vi "String to Magnet device cluster.vi"(11 "Magnet Device Details":string="VTRT:0:STAT:0:NICK:GRPN:BIPL:ON:MAN:HVER::FVER::SERL::ATOB:1.0:SWPR:None:SHTC:100.0:VLIM:10.00:IND:1:CLIM:10.0:ACTN:CLMP:SIG:CURR:0.0000A:PCUR:0.0000A:VOLT:0.0000V:RCST:0.0000A/m:RFST:0.0000T/m:SWHN:OFF:FSET:0.0000T:FLD:0.0000T:RFLD:1200.0000T/min:CSET:0.0000A:RCUR:1200.0000A/min:PFLD:0.0000T:SWHT:OFF:OCNF:PARA") -> (3 "Magnet PSU":T1={"Manufacturing"={"Hardware Version"="", "Firmware Version"="", "Serial Number"=""}, "Nickname"="", "Bipolar Output"="", "String"="SERS", "Current Limit"=0.0, "AtoB"=0.0, "Inductance"=0.0, "Switch Present"="", "Swh Htr Current"=0.0, "SW VLIM"=0.0, "V Trans Time"=0.0, "Magnet PSU Signals"={"Voltage"=0.0, "Current"=0.0, "Current Rate"=0.0, "Field"=0.0, "Field Rate"=0.0, "Persistant Current"=0.0, "Persistant Field"=0.0, "Target Current"=0.0, "Target Field"=0.0, "Target Current Rate"=0.0, "Target Field Rate"=0.0, "Switch Heater Status (SWHT)"="", "Switch Heater Status (SWHN)"=""}, "PSU Action"="SERS", "Status"="", "Level Limit"=0.0, "Temperature Limit"=0.0} {"Temperature Limit" format="%#.1f"; "Level Limit" format="%#.1f"; "V Trans Time" format="%#.1f"; "SW VLIM" format="%#.1f"; "Swh Htr Current" format="%#.1f"; "Inductance" format="%#.1f"; "AtoB" format="%#.1f"; "Current Limit" format="%#.1f"})   [LabVIEW 2018, in "Mercury iXX.lvlib" / "Magnet.lvlib"]
uses:
  Magnet.lvlib
  Device (Read).ctl
  Manufacturing Data.ctl
  Signals (Read).ctl
  Mercury iXX.lvlib
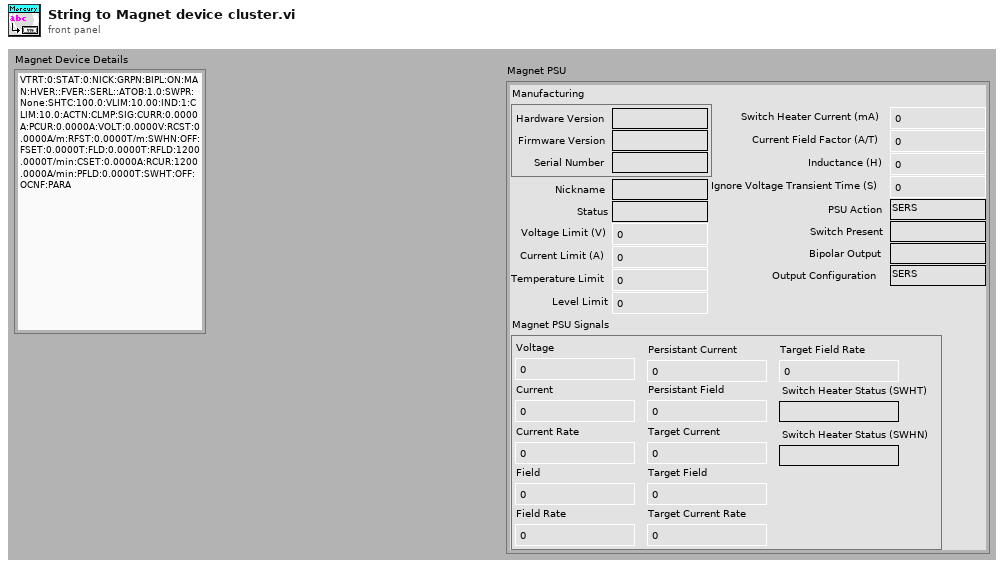
[diagram p1: front panel]
types:
  T1 = typedef "Mercury iXX.lvlib/Magnet.lvlib/Device (Read).ctl" = cluster{"Manufacturing":T2, "Nickname":string, "Bipolar Output":string, "String":string, "Current Limit":dbl, "AtoB":dbl, "Inductance":dbl, "Switch Present":string, "Swh Htr Current":dbl, "SW VLIM":dbl, "V Trans Time":dbl, "Magnet PSU Signals":T3, "PSU Action":string, "Status":string, "Level Limit":dbl, "Temperature Limit":dbl}
  T2 = typedef "Mercury iXX.lvlib/Manufacturing Data.ctl" = cluster{"Hardware Version":string, "Firmware Version":string, "Serial Number":string}
  T3 = typedef "Mercury iXX.lvlib/Magnet.lvlib/Signals (Read).ctl" = cluster{"Voltage":dbl, "Current":dbl, "Current Rate":dbl, "Field":dbl, "Field Rate":dbl, "Persistant Current":dbl, "Persistant Field":dbl, "Target Current":dbl, "Target Field":dbl, "Target Current Rate":dbl, "Target Field Rate":dbl, "Switch Heater Status (SWHT)":string, "Switch Heater Status (SWHN)":string}
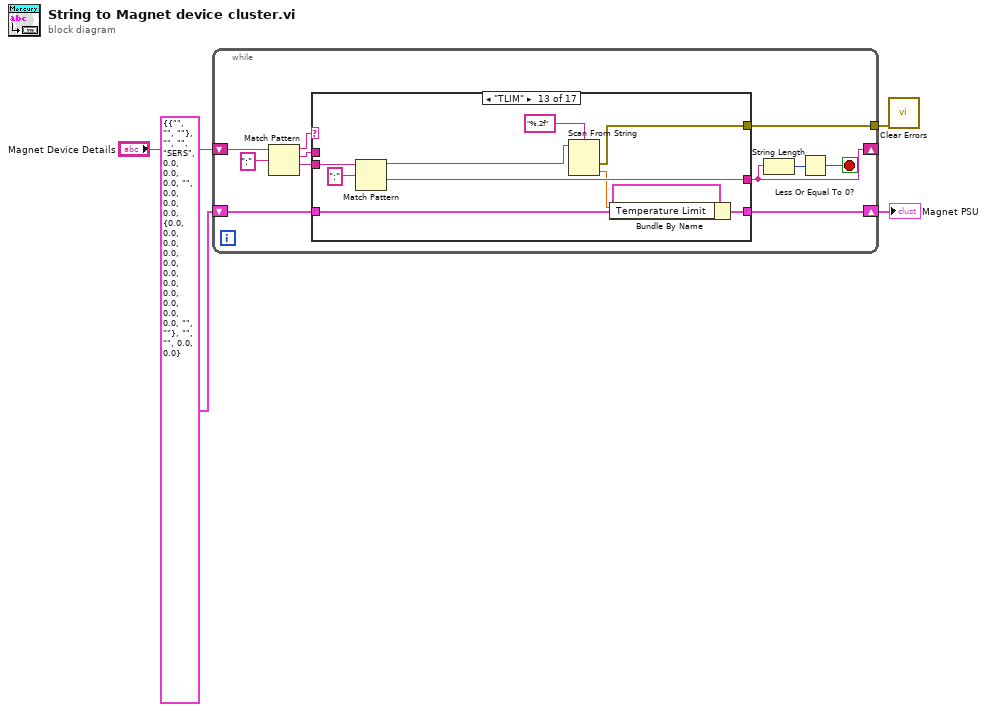
[diagram p0: block diagram]
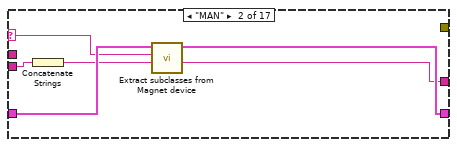
[diagram p3: hidden frame]
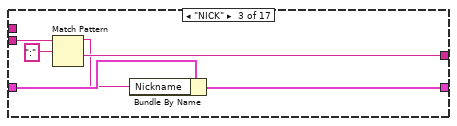
[diagram p4: hidden frame]
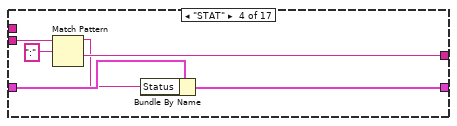
[diagram p5: hidden frame]
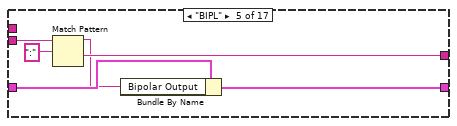
[diagram p6: hidden frame]
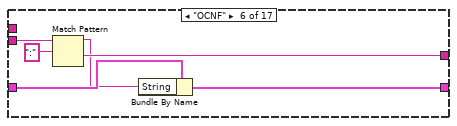
[diagram p7: hidden frame]
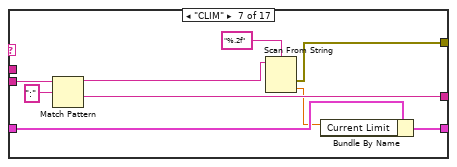
[diagram p8: hidden frame]
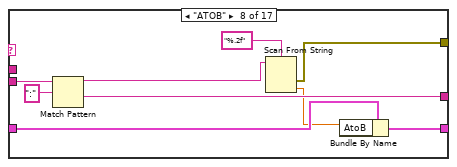
[diagram p9: hidden frame]
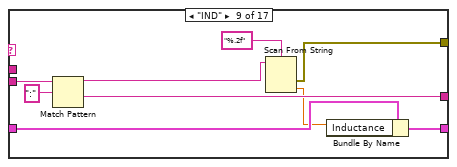
[diagram p10: hidden frame]
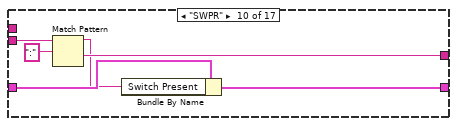
[diagram p11: hidden frame]
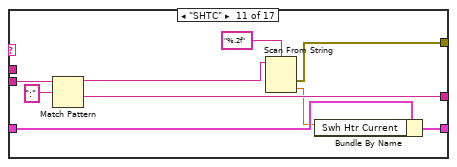
[diagram p12: hidden frame]
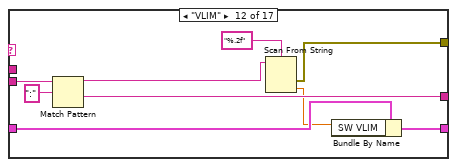
[diagram p13: hidden frame]
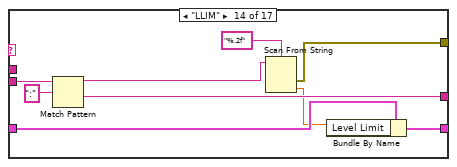
[diagram p14: hidden frame]
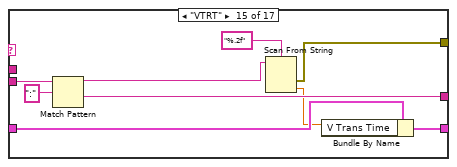
[diagram p15: hidden frame]
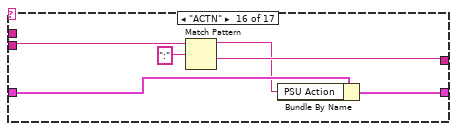
[diagram p16: hidden frame]
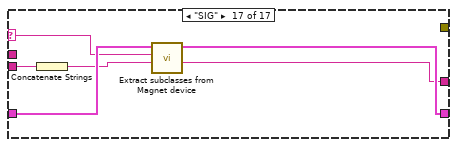
[diagram p17: hidden frame]
diagram:
  n1 = while {
    shift-right: [w11] -> w3
    shift-left: T1 {"Manufacturing"={"Hardware Version"="", "Firmware Version"="", "Serial Number"=""}, "Nickname"="", "Bipolar Output"="", "String"="SERS", "Current Limit"=0.0, "AtoB"=0.0, "Inductance"=0.0, "Switch Present"="", "Swh Htr Current"=0.0, "SW VLIM"=0.0, "V Trans Time"=0.0, "Magnet PSU Signals"={"Voltage"=0.0, "Current"=0.0, "Current Rate"=0.0, "Field"=0.0, "Field Rate"=0.0, "Persistant Current"=0.0, "Persistant Field"=0.0, "Target Current"=0.0, "Target Field"=0.0, "Target Current Rate"=0.0, "Target Field Rate"=0.0, "Switch Heater Status (SWHT)"="", "Switch Heater Status (SWHN)"=""}, "PSU Action"="", "Status"="", "Level Limit"=0.0, "Temperature Limit"=0.0} ("Magnet PSU") -> [w12]
    shift-right: [w7] -> _
    shift-left: "Magnet Device Details" -> [w14]
    tunnel: [w5] -> w1
    stop <- w6 stop-if-true
    n2 = Match Pattern(string=w14, regular expression=":") -> (before substring=w13:string, match substring=w10:string, after substring=w9:string)  [unwired: 2 out]
    n3 = case shown="\"TLIM\"" w13 {
      selector: w13 -> [_ w22 _ _ _ _ _ _ _ _ _ _ _ _ _ _ w135]
      tunnel: w10 -> [_ _ _ _ _ _ _ _ _ _ _ _ _ _ _ _ _]
      tunnel: w12 -> [w17 w23 w27 w33 w39 w45 w54 w63 w72 w78 w87 w96 w105 w114 w123 w128 w136]
      tunnel: [w17 w21 w26 w32 w38 w44 w53 w62 w71 w77 w86 w95 w104 w113 w122 w127 w133] -> w11
      tunnel: [w16 w20 w25 w31 w37 w43 w51 w60 w69 w76 w84 w93 w102 w111 w120 w129 w132] -> w7
      tunnel: w9 -> [w16 w19 w28 w34 w40 w46 w55 w64 w73 w79 w88 w97 w106 w115 w124 w130 w137]
      tunnel: [_ _ _ _ _ _ w48 w57 w66 _ w81 w90 w99 w108 w117 _ _] -> w5
      frame "", Default {
      }
      frame "MAN" {
        n4 = Concatenate Strings(w19) -> (w18:string)
        n5 = call "Extract subclasses from Magnet device.vi"("Data In"=w18, "Class"=w22, "Aux Device Settings in"=w23) -> ("Data out"=w20:string, "Aux Device Settings out"=w21:T1)  [unwired: 7 out]
      }
      frame "NICK" {
        n6 = Match Pattern(string=w28, regular expression=":") -> (before substring=w24:string, after substring=w25:string)  [unwired: 3 out]
        n7 = Bundle By Name(cluster=w27, "Nickname"=w24) -> (w26:T1)
      }
      frame "STAT" {
        n8 = Match Pattern(string=w34, regular expression=":") -> (before substring=w30:string, after substring=w31:string)  [unwired: 3 out]
        n9 = Bundle By Name(cluster=w33, "Status"=w30) -> (w32:T1)
      }
      frame "BIPL" {
        n10 = Match Pattern(string=w40, regular expression=":") -> (before substring=w36:string, after substring=w37:string)  [unwired: 3 out]
        n11 = Bundle By Name(cluster=w39, "Bipolar Output"=w36) -> (w38:T1)
      }
      frame "OCNF" {
        n12 = Match Pattern(string=w46, regular expression=":") -> (before substring=w42:string, after substring=w43:string)  [unwired: 3 out]
        n13 = Bundle By Name(cluster=w45, "String"=w42) -> (w44:T1)
      }
      frame "CLIM" {
        n14 = Match Pattern(string=w55, regular expression=":") -> (before substring=w52:string, after substring=w51:string)  [unwired: 3 out]
        n15 = Scan From String(format string="%.2f", input string=w52) -> (error out=w48:errorcluster, output 1=w50:dbl)  [unwired: 2 in, 3 out]
        n16 = Bundle By Name(cluster=w54, "Current Limit"=w50) -> (w53:T1)
      }
      frame "ATOB" {
        n17 = Match Pattern(string=w64, regular expression=":") -> (before substring=w61:string, after substring=w60:string)  [unwired: 3 out]
        n18 = Scan From String(format string="%.2f", input string=w61) -> (error out=w57:errorcluster, output 1=w59:dbl)  [unwired: 2 in, 3 out]
        n19 = Bundle By Name(cluster=w63, "AtoB"=w59) -> (w62:T1)
      }
      frame "IND" {
        n20 = Match Pattern(string=w73, regular expression=":") -> (before substring=w70:string, after substring=w69:string)  [unwired: 3 out]
        n21 = Scan From String(format string="%.2f", input string=w70) -> (error out=w66:errorcluster, output 1=w68:dbl)  [unwired: 2 in, 3 out]
        n22 = Bundle By Name(cluster=w72, "Inductance"=w68) -> (w71:T1)
      }
      frame "SWPR" {
        n23 = Match Pattern(string=w79, regular expression=":") -> (before substring=w75:string, after substring=w76:string)  [unwired: 3 out]
        n24 = Bundle By Name(cluster=w78, "Switch Present"=w75) -> (w77:T1)
      }
      frame "SHTC" {
        n25 = Match Pattern(string=w88, regular expression=":") -> (before substring=w85:string, after substring=w84:string)  [unwired: 3 out]
        n26 = Scan From String(format string="%.2f", input string=w85) -> (error out=w81:errorcluster, output 1=w83:dbl)  [unwired: 2 in, 3 out]
        n27 = Bundle By Name(cluster=w87, "Swh Htr Current"=w83) -> (w86:T1)
      }
      frame "VLIM" {
        n28 = Match Pattern(string=w97, regular expression=":") -> (before substring=w94:string, after substring=w93:string)  [unwired: 3 out]
        n29 = Scan From String(format string="%.2f", input string=w94) -> (error out=w90:errorcluster, output 1=w92:dbl)  [unwired: 2 in, 3 out]
        n30 = Bundle By Name(cluster=w96, "SW VLIM"=w92) -> (w95:T1)
      }
      frame "TLIM" {
        n31 = Match Pattern(string=w106, regular expression=":") -> (before substring=w103:string, after substring=w102:string)  [unwired: 3 out]
        n32 = Scan From String(format string="%.2f", input string=w103) -> (error out=w99:errorcluster, output 1=w101:dbl)  [unwired: 2 in, 3 out]
        n33 = Bundle By Name(cluster=w105, "Temperature Limit"=w101) -> (w104:T1)
      }
      frame "LLIM" {
        n34 = Match Pattern(string=w115, regular expression=":") -> (before substring=w112:string, after substring=w111:string)  [unwired: 3 out]
        n35 = Scan From String(format string="%.2f", input string=w112) -> (error out=w108:errorcluster, output 1=w110:dbl)  [unwired: 2 in, 3 out]
        n36 = Bundle By Name(cluster=w114, "Level Limit"=w110) -> (w113:T1)
      }
      frame "VTRT" {
        n37 = Match Pattern(string=w124, regular expression=":") -> (before substring=w121:string, after substring=w120:string)  [unwired: 3 out]
        n38 = Scan From String(format string="%.2f", input string=w121) -> (error out=w117:errorcluster, output 1=w119:dbl)  [unwired: 2 in, 3 out]
        n39 = Bundle By Name(cluster=w123, "V Trans Time"=w119) -> (w122:T1)
      }
      frame "ACTN" {
        n40 = Match Pattern(string=w130, regular expression=":") -> (before substring=w126:string, after substring=w129:string)  [unwired: 3 out]
        n41 = Bundle By Name(cluster=w128, "PSU Action"=w126) -> (w127:T1)
      }
      frame "SIG" {
        n42 = Concatenate Strings(w137) -> (w134:string)
        n43 = call "Extract subclasses from Magnet device.vi"("Data In"=w134, "Class"=w135, "Aux Device Settings in"=w136) -> ("Data out"=w132:string, "Aux Device Settings out"=w133:T1)  [unwired: 7 out]
      }
    }
    n44 = String Length(string=w7) -> (length=w8:i32)
    n45 = Less Or Equal To 0?(x=w8) -> (x <= 0?=w6:bool)
  }
  "Magnet PSU" <- w3
  n46 = call "Clear Errors.vi"("error in (no error)"=w1) -> ()  [unwired: 1 in, 6 out]
